vi "Exemple_Metrics_Zero_One_Loss.vi"() -> ()   [LabVIEW 2020]
uses:
  Objet/3 - Model selection and evaluation/3.3 - Metrics and scoring/zero_one_loss/Zero_One_Loss.vi
panel:
  out "Score":string
  out "error out":errorcluster caption="sortie d'erreur"
  in  "error in (no error)":errorcluster caption="entrée d'erreur (pas d'erreur)"
  in  "zero_one_loss":cluster{"normalize":bool, "sample_weight":dbl[]}={"normalize"=TRUE, "sample_weight"=[]}
  in  "y_pred":string[][](array[string])=[["1"], ["2"], ["3"], ["4"]]
  in  "y_true":string[][](array[string])=[["2"], ["2"], ["3"], ["4"]]
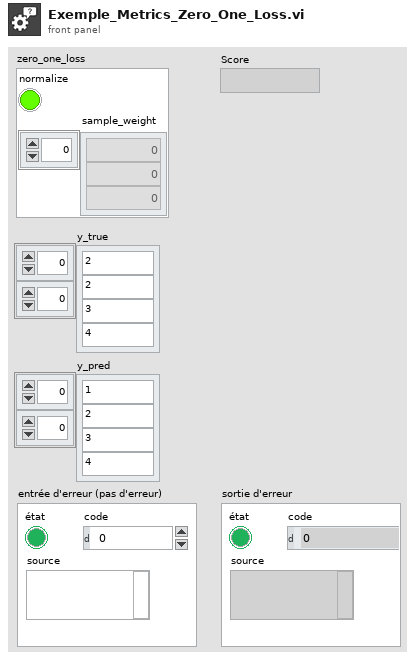
[diagram p1: front panel]
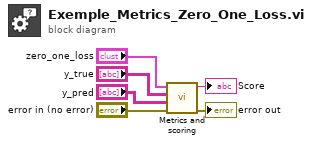
[diagram p0: block diagram]
diagram:
  n1 = call-poly "Metrics and scoring.vi"("error in (no error)"="error in (no error)", "y_pred"="y_pred", "y_true"="y_true", "zero_one_loss"="zero_one_loss") -> ("error out"=→"error out":errorcluster, "Score"=→"Score":string)  [unwired: 6 in]
